vi "stopButton.vi"() -> ()   [LabVIEW 2011]
panel:
  out "stopsignal":bool
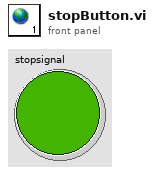
[diagram p1: front panel]
diagram:
